vi "PH_AxisGUI_6P.set GUI Refs.vi"(0 "i ref in":refnum<vi>, 2 "Class":string, 3 "GUI Refs":cluster{"Axis GUI Base Class Refs":T1[]}, 4 "AxisSelection":refnum<vi>, 5 "error in":errorcluster) -> (14 "i ref out":refnum<vi>, 19 "error out":errorcluster)   [LabVIEW 2014, in "PH_AxisGUI_6P.lvlib"]
doc: "This VI is forseen to set the GUI element references; it shall be used especially within child classes."
uses:
  PH_AxisGUI_6P.lvlib
  PH_Basics/PH_AxisGUI_BaseClass/PH_AxisGUI_BaseClass.Axis GUI Refs.ctl
  PH_Basics/PH_Stepmotor_BaseClass/PH_Stepmotor_BaseClass.Axis Address.ctl
  PH_Basics/PH_Stepmotor_BaseClass/PH_Stepmotor_BaseClass.Axis Settings.ctl
  PH_Basics/PH_Stepmotor_BaseClass/PH_Stepmotor_BaseClass.Motor Type.ctl
  PH_Basics/PH_Stepmotor_BaseClass/PH_Stepmotor_BaseClass.Axis Activity.ctl
  PH_Basics/PH_AxisGUI_BaseClass/PH_AxisGUI_BaseClass.lvlib
  PH_Basics/PH_Stepmotor_BaseClass/PH_Stepmotor_BaseClass.lvlib
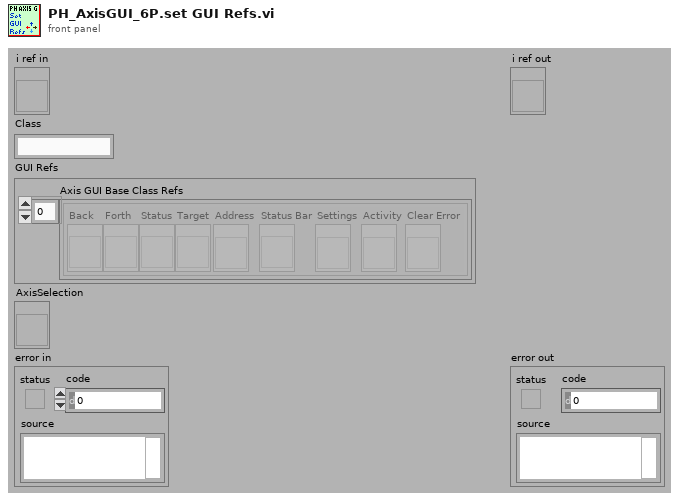
[diagram p1: front panel]
types:
  T1 = typedef "PH_AxisGUI_BaseClass.lvlib/PH_AxisGUI_BaseClass.Axis GUI Refs.ctl" = cluster{"Back":refnum<vi>, "Forth":refnum<vi>, "Status":refnum<vi>, "Target":refnum<vi>, "Address":refnum<vi>, "Status Bar":refnum<vi>, "Settings":refnum<vi>, "Activity":refnum<vi>, "Clear Error":refnum<vi>}
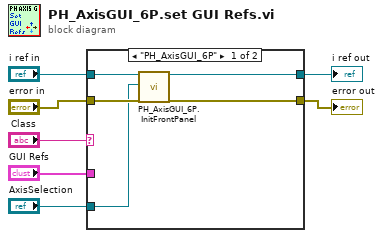
[diagram p0: block diagram]
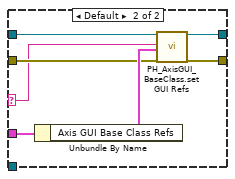
[diagram p2: hidden frame]
diagram:
  n1 = case shown="\"PH_AxisGUI_6P\"" "Class" {
    selector: "Class" -> [_ w13]
    tunnel: "GUI Refs" -> [_ w19]
    tunnel: "i ref in" -> [w12 w18]
    tunnel: "error in" -> [w11 w16]
    tunnel: [w9 w15] -> w4
    tunnel: [w8 w14] -> w3
    tunnel: "AxisSelection" -> [w10 _]
    frame "PH_AxisGUI_6P" {
      n2 = call "PH_AxisGUI_6P.InitFrontPanel.vi"("i ref in"=w12, "AxisSelection"=w10, "error in"=w11) -> ("i ref out"=w9:refnum<vi>, "error out"=w8:errorcluster)  [unwired: 15 in]
    }
    frame Default {
      n3 = Unbundle By Name(w19) -> ("Axis GUI Base Class Refs"=w17:T1[])
      n4 = call "PH_AxisGUI_BaseClass.set GUI Refs.vi"("i ref in"=w18, "Class"=w13, "Axis GUI Base Class Refs"=w17, "error in"=w16) -> ("i ref out"=w15:refnum<vi>, "error out"=w14:errorcluster)  [unwired: 14 in]
    }
  }
  "error out" <- w3
  "i ref out" <- w4
